vi "_getInstallationResults.vi"(8 "error in (no error)":errorcluster, 11 "Item Names":string[][](array[string])) -> (0 "error out":errorcluster)   [LabVIEW 2017]
panel:
  in  "OK":bool
  out "Multicolumn Listbox":i32(listbox)
  # "Results of the installation:"
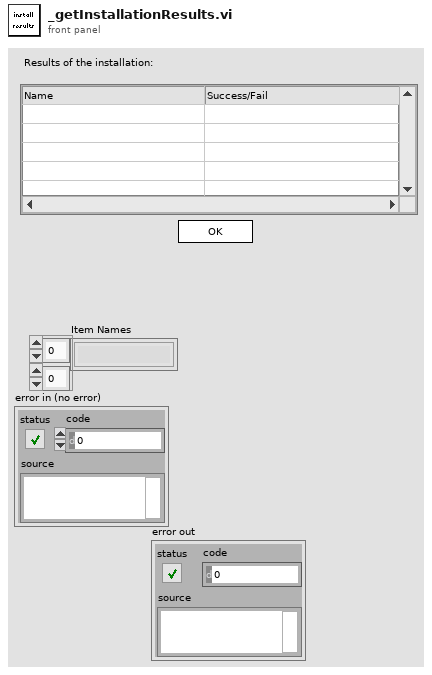
[diagram p1: front panel]
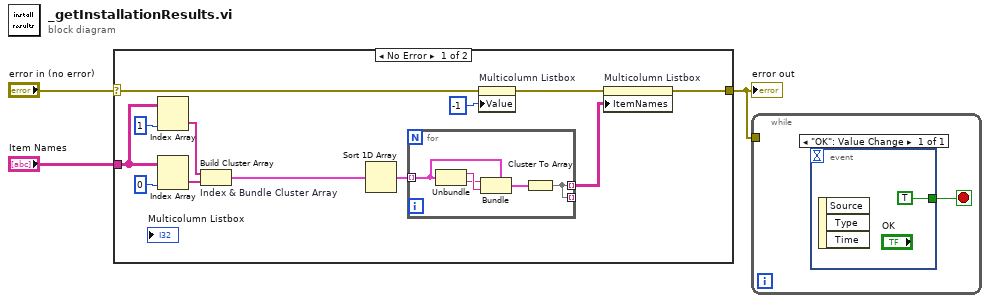
[diagram p0: block diagram]
diagram:
  n1 = case shown="No Error" "error in (no error)" {
    selector: "error in (no error)" -> [w4 w21]
    tunnel: "Item Names" -> [w14 _]
    tunnel: [w5 w21] -> w2
    frame No Error {
      n2 = Index Array(array=w14, index (col)=1 ("disabled index (col)")) -> (element=w12:string[])  [unwired: 1 in]
      n3 = Index Array(array=w14, index (col)=0 ("disabled index (col)")) -> (element=w11:string[])  [unwired: 1 in]
      n4 = Build Cluster Array "Index & Bundle Cluster Array"(w12, w11) -> (w10:cluster{string, string}[])
      n5 = Sort 1D Array(array=w10) -> (sorted array=w9:cluster{string, string}[])
      n6 = for {
        tunnel: w9 -> [w20] mode=indexing
        tunnel: [w16] -> _ mode=indexing
        tunnel: [w16] -> w8 mode=indexing
        n7 = Unbundle(w20) -> (w19:string, w18:string)
        n8 = Bundle(cluster=w20, w18, w19) -> (w17:cluster{string, string})
        n9 = Cluster To Array(cluster=w17) -> (array=w16:string[])
      }
      n10 = property on="Multicolumn Listbox" class="MCListbox (strict)"(error in=w4, "Value"=-1 ("Multicolumn Listbox")) -> (error out=w6:errorcluster)  [unwired: 1 in, 1 out]
      n11 = property on="Multicolumn Listbox" class="MCListbox (strict)"(error in=w6, "ItemNames"=w8) -> (error out=w5:errorcluster)  [unwired: 1 in, 1 out]
    }
    frame Error {
    }
  }
  "error out" <- w2
  n12 = while {
    tunnel: w2 -> [_]
    stop <- w22 stop-if-true
    n13 = event shown="[0] \"OK\": Value Change" {
      selector: _ -> [_]
      dyn-events: _ -> [_]
      timeout: _ -> [_]
      tunnel: [TRUE] -> w22
      event "OK": Value Change {
        n14 = event-data() -> ()  [unwired: 1 in, 3 out]
      }
    }
  }
